vi "Initialise.vi"() -> (0 "error out":errorcluster, 3 "Launcher Actor out":refnum<class "Launcher Actor.lvclass">, 5 "Actor":refnum<event-registration>)   [LabVIEW 2021, in "Launcher Actor.lvclass"]
uses:
  Launcher Actor.lvclass
  Launcher Actor.lvclass/Launcher Actor.ctl
  C:/dev/LabVIEW/LabMelee/Source/Re-use Libraries/Minimal Actor Framework/Actors/Base Actor/Actor/Actor.lvclass
  C:/dev/LabVIEW/LabMelee/Source/Application Specific/Actors/Launcher/Actor/Launcher Actor.lvclass
  Main Controller/Actor/Main Controller Actor.lvclass
  Re-use Libraries/Minimal Actor Framework/Actors/Base Actor/API/Actor API.lvclass
  Globals.vi
  Re-use Libraries/Minimal Actor Framework/Messaging/Messenger/Messenger.lvclass
  Re-use Libraries/Minimal Actor Framework/Actors/Base Actor/Actor/Front Panel State.ctl
  Re-use Libraries/Minimal Actor Framework/Actors/Base Actor/Actor/Actor.lvclass
  Re-use Libraries/Application Info/App Info.lvlib
  Re-use Libraries/Utility/Utility.lvlib
  <userlib>/_OpenG.lib/appcontrol/appcontrol.llb/openg_application_control.lvlib
  Main INI/Main INI.lvlib
  Process.vi
  Re-use Libraries/Minimal Actor Framework/Messaging/Message/Message.lvclass
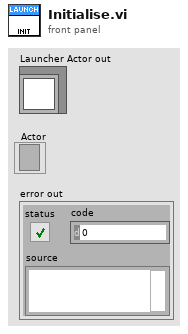
[diagram p1: front panel]
types:
  T1 = typedef "Actor.lvclass/Front Panel State.ctl" = enum32{"Invalid", "Standard", "Closed", "Hidden", "Minimized", "Maximized"}
  T2 = enum32{"invalid app kind", "Development System", "Run Time System", "Student Edition", "Embedded LabVIEW", "Evaluation", "Custom"}
  T3 = typedef "Utility.lvlib/App Paths.ctl" = cluster{"App Ini File":path, "App Data Dir":path, "Config Dir":path, "App Root Dir":path}
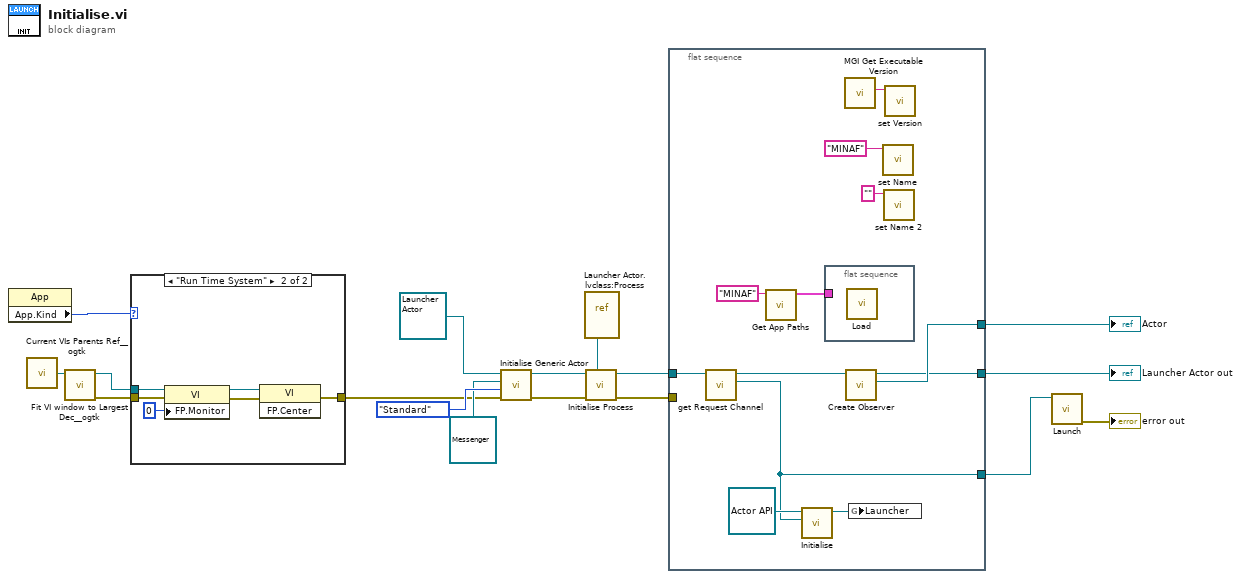
[diagram p0: block diagram]
diagram:
  n1 = property class="App"() -> ("App.Kind"=w9:T2)  [unwired: 2 in, 2 out]
  n2 = call <userlib>:"Current VIs Parents Ref__ogtk.vi"() -> ("Calling VI's Reference"=w10:refnum<vi>)  [unwired: 2 in]
  n3 = call <userlib>:"Fit VI window to Largest Dec__ogtk.vi"("VI Ref (calling VI)"=w10) -> ("error out"=w6:errorcluster, "dup VI Ref"=w8:refnum<vi>)  [unwired: 5 in]
  n4 = case shown="\"Run Time System\"" w9 {
    tunnel: w8 -> [_ w24]
    tunnel: [w18 w21] -> w7
    tunnel: w6 -> [w18 w19]
    frame "invalid app kind", Default {
    }
    frame "Run Time System" {
      n5 = property class="VI"(reference=w24, error in=w19, "FP.Monitor"=u16 0 ("Front Panel Window:Monitor")) -> (reference out=w22:refnum<vi>, error out=w20:errorcluster)
      n6 = invoke class="VI" method="FP.Center"(reference=w22, error in=w20) -> (error out=w21:errorcluster)  [unwired: 1 in, 2 out]
    }
  }
  n7 = call-dynamic "Initialise Generic Actor.vi"("error in (no error)"=w7, "Front Panel State"=Front_Panel_State."Standard", "Response Channel"=refnum<class "Messenger.lvclass"> refnum, "Actor in"=refnum<class "Launcher Actor.lvclass"> refnum ("Launcher Actor.lvclass")) -> ("error out"=w2:errorcluster, "Actor out"=w5:refnum<class "Launcher Actor.lvclass">)  [unwired: 6 in]
  n8 = vi-ref "Launcher Actor.lvclass:Process.vi"() -> (w3:refnum<vi>)
  n9 = call-dynamic "Initialise Process.vi"("Process"=w3, "error in (no error)"=w2, "Actor in"=w5) -> ("error out"=w1:errorcluster, "Actor out"=w4:refnum<class "Launcher Actor.lvclass">)  [unwired: 7 in]
  n10 = flat-sequence {
    tunnel: [w29] -> w12
    tunnel: w4 -> [w34]
    tunnel: [w30] -> w13
    tunnel: [w28] -> w11
    tunnel: w1 -> [_]
    frame #0 {
      n11 = call "get Request Channel.vi"("Actor in"=w34) -> ("Request Channel"=w28:refnum<class "Messenger.lvclass">, "Actor out"=w31:refnum<class "Launcher Actor.lvclass">)  [unwired: 8 in, 1 out]
      n12 = call "Get App Paths.vi"("Build Name"="MINAF" ("Name")) -> ("Paths"=w25:T3)  [unwired: 9 in, 1 out]
      n13 = call "Initialise.vi"("Request Channel"=w28, "Actor API in"=refnum<class "Actor API.lvclass"> refnum ("Actor API.lvclass")) -> ("Actor API out"=w32:refnum<class "Actor API.lvclass">)  [unwired: 8 in, 1 out]
      n14 = flat-sequence {
        tunnel: w25 -> [_]
        frame #0 {
          n15 = call "Load.vi"() -> ()  [unwired: 10 in, 2 out]
        }
      }
      n16 = call <userlib>:"MGI Get Executable Version.vi"() -> ("Version"=w27:string)  [unwired: 7 in]
      n17 = call-dynamic "Create Observer.vi"("Actor in"=w31) -> ("Actor"=w30:refnum<event-registration>, "Actor out"=w29:refnum<class "Launcher Actor.lvclass">)  [unwired: 8 in, 1 out]
      n18 = global write "Globals.vi" "Launcher"(w32) -> ()
      n19 = call "set Name.vi"("Name"="MINAF") -> ()  [unwired: 10 in, 1 out]
      n20 = call "set Name 2.vi"("Name 2"="") -> ()  [unwired: 10 in, 1 out]
      n21 = call "set Version.vi"("Version"=w27) -> ()  [unwired: 10 in, 1 out]
    }
  }
  n22 = call "Launch.vi"("Response Channel"=w11) -> ("error out"=→"error out":errorcluster)  [unwired: 10 in]
  "Launcher Actor out" <- w12
  "Actor" <- w13
